vi "Get Default Data from TD.vi"(8 "error in (no error)":errorcluster, 10 "Type Descriptor":refnum<class "TD.lvclass">) -> (0 "error out":errorcluster, 2 "Default VData":refnum<class "variant.lvclass">)   [LabVIEW 2020, in "variant.lvlib" / "variant.lvclass"]
doc: "Returns default data of the type defined by the TD. This VI calls itself recursively.\n\nThis VI is <b>Reentrant</b>"
uses:
  variant.lvclass
  variant.lvclass/variant.ctl
  <userlib>/_OpenG.lib/error/error.llb/openg_error.lvlib
  TD.lvclass
  Bytes/Bytes.lvclass
  DataString/DataString.lvclass
  C:/projects/OpenG-Variant-Data-Library/source/library/Bytes/Bytes.lvclass
  C:/projects/OpenG-Variant-Data-Library/source/library/LVData/DataString/DataString.lvclass
panel:
  # "Please visit http://www.OpenG.org to learn about the\nOpen Source LabVIEW software movement.\n\nNOTICE -- YOU MUST LEAVE THIS NOTICE IN PLACE.  PER THE TERMS OF THE LICENSE BELOW, YOU MAY SUBLICENSE THIS SOFTWARE \nIN ANY WAY THAT DOES NOT CONFLICT WITH THIS LICENSE.\n\n### BSD License (http://www.opensource.org/licenses/bsd-license.php) Begin ###\n \nCopyright (c) 2002, Jean-Pierre Drolet <drolet_jp@hotmail.com>\nCopyright (c) 2002-2006, Jim Kring <jim@jimkring.com>\nCopyright (c) 2011, Jonathon Green <jg@jgcode.net>\n\nAll rights reserved.\n\nRedistribution and use in source and binary forms, with or without modification, are permitted provided that the following conditions are met:\n\n    * Redistributions of source code must retain the above copyright notice, this list of conditions and the following disclaimer.\n    * Redistributions in binary form must reproduce the above copyright notice, this list of conditions and the following disclaimer in the \n       documentation and/or other materials provided with the distribution.\n    * Neither the name of SciWare, James Kring, Inc., nor the names of its contributors may be used to endorse or promote products derived \n       from this software without specific prior written permission.\n\nTHIS SOFTWARE IS PROVIDED BY THE COPYRIGHT HOLDERS AND CONTRIBUTORS \"AS IS\" AND ANY EXPRESS OR IMPLIED WARRANTIES, \nINCLUDING, BUT NOT LIMITED TO, THE IMPLIED WARRANTIES OF MERCHANTABILITY AND FITNESS FOR A PARTICULAR PURPOSE ARE \nDISCLAIMED. IN NO EVENT SHALL THE COPYRIGHT OWNER OR CONTRIBUTORS BE LIABLE FOR ANY DIRECT, INDIRECT, INCIDENTAL,\n SPECIAL, EXEMPLARY, OR CONSEQUENTIAL DAMAGES (INCLUDING, BUT NOT LIMITED TO, PROCUREMENT OF SUBSTITUTE GOODS OR \nSERVICES; LOSS OF USE, DATA, OR PROFITS; OR BUSINESS INTERRUPTION) HOWEVER CAUSED AND ON ANY THEORY OF LIABILITY, \nWHETHER IN CONTRACT, STRICT LIABILITY, OR TORT (INCLUDING NEGLIGENCE OR OTHERWISE) ARISING IN ANY WAY OUT OF THE USE \nOF THIS SOFTWARE, EVEN IF ADVISED OF THE POSSIBILITY OF SUCH DAMAGE.\n\n### BSD License End ###"
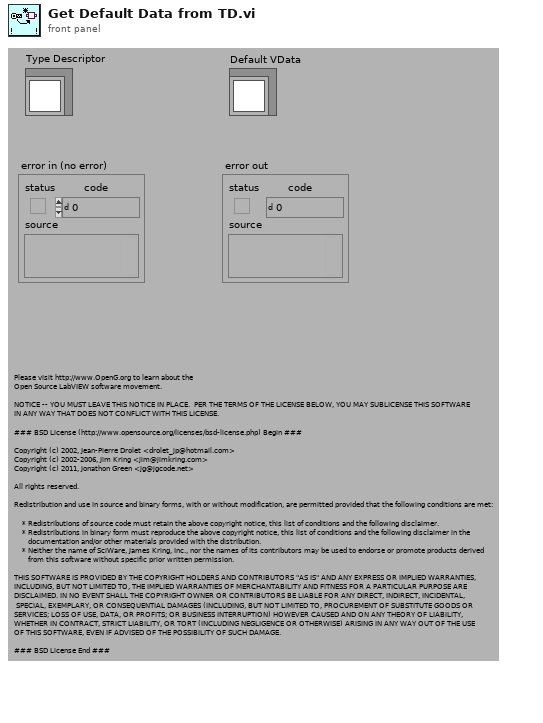
[diagram p1: front panel]
types:
  T1 = typedef "openg_variant.lvlib/Type Descriptor Enumeration.ctl" = enum8{"<Null>", "I8", "I16", "I32", "I64", "U8", "U16", "U32", "U64", "SGL", "DBL", "EXT", "CSG", "CDB", "CXT", "0x0F", "0x10", "0x11", "0x12", "0x13", "0x14", "Enum U8", "Enum U16", "Enum U32", "Enum U64", "SGL PQ", "DBL PQ", "EXT PQ", "CSG PQ", "CDB PQ", "CXT PQ", "0x1F", "0x20", "Boolean", "0x22", "0x23", "0x24", "0x25", "0x26", "0x27", "0x28", "0x29", "0x2A", "0x2B", "0x2C", "0x2D", "0x2E", "0x2F", "String", "0x31", "Path", "Pict", "0x34", "0x35", "0x36", "DAQ", "0x38", "0x39", "0x3A", "0x3B", "0x3C", "0x3D", "0x3E", "0x3F", "Array", "0x41", "0x42", "0x43", "0x44", "0x45", "0x46", "0x47", "0x48", "0x49", "0x4A", "0x4B", "0x4C", "0x4D", "0x4E", "0x4F", "Cluster", "0x51", "0x52", "Variant", "Waveform", "0x55", "0x56", "0x57", "0x58", "0x59", "0x5A", "0x5B", "0x5C", "0x5D", "0x5E", "Fixed Point", "0x60", "0x61", "0x62", "0x63", "0x64", "0x65", "0x66", "0x67", "0x68", "0x69", "0x6A", "0x6B", "0x6C", "0x6D", "0x6E", "0x6F", "Refnum", "0x71", "0x72", "Set Collection", "Map Collection"}
  T2 = typedef "openg_variant.lvlib/Waveform Subtype Enum.ctl" = enum8{"<Not a Waveform Type>", "0x01", "Analog 16-bit signed", "Analog Double-Precision", "0x04", "Analog Single Precision", "Timestamp", "Digital Data", "Digital Waveform", "Dynamic Data", "Analog Extended-Precision", "Analog 8-bit unsigned", "Analog 16-bit unsigned", "Analog 32-bit unsigned", "Analog 8-bit signed", "Analog 32-bit signed", "Analog Complex Single-Precision", "Analog Complex Double-Precision", "Analog Complex Extended Precision", "Analog 64-bit signed", "Analog 64-bit unsigned"}
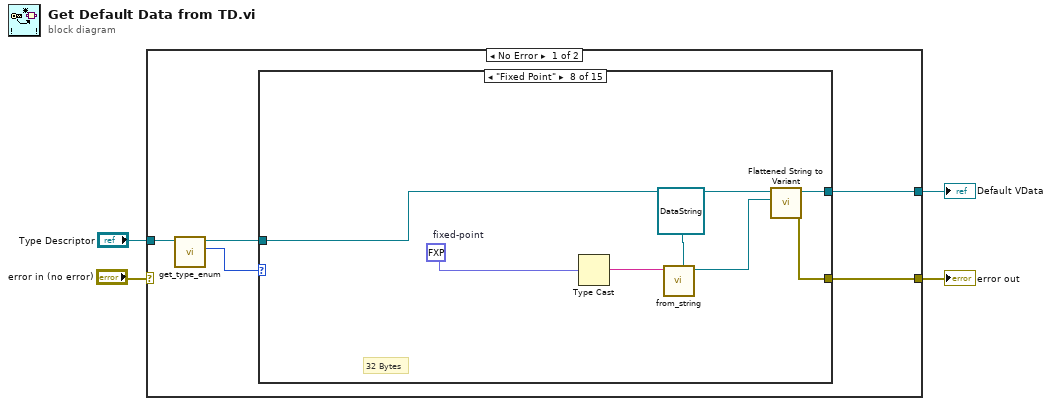
[diagram p0: block diagram]
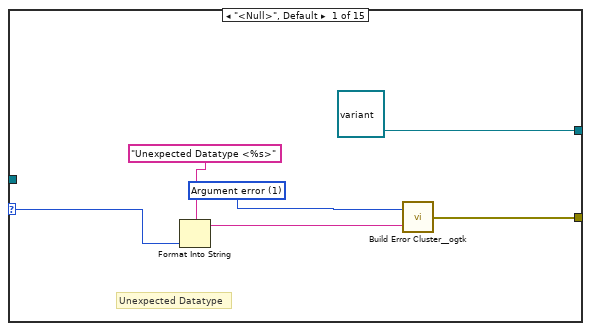
[diagram p2: hidden frame]
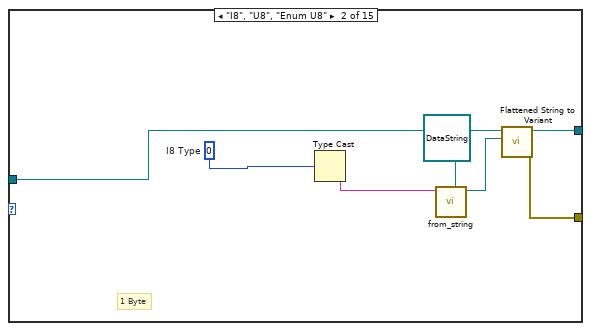
[diagram p3: hidden frame]
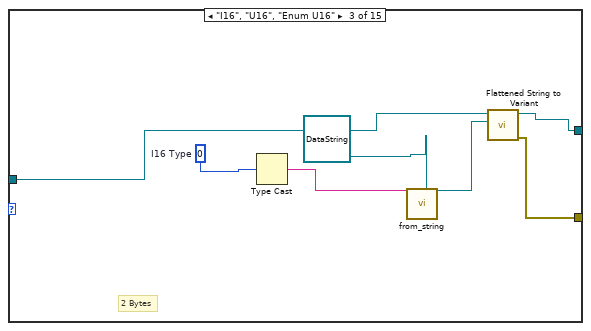
[diagram p4: hidden frame]
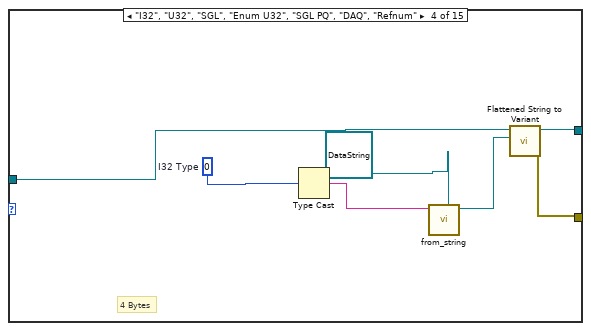
[diagram p5: hidden frame]
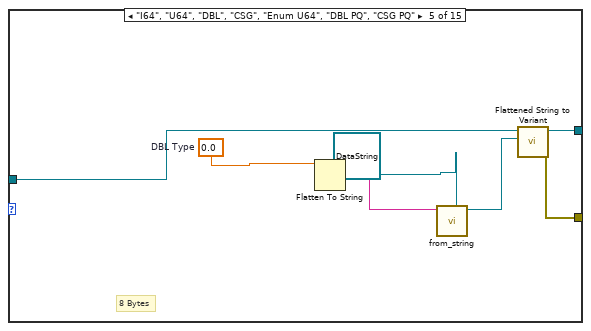
[diagram p6: hidden frame]
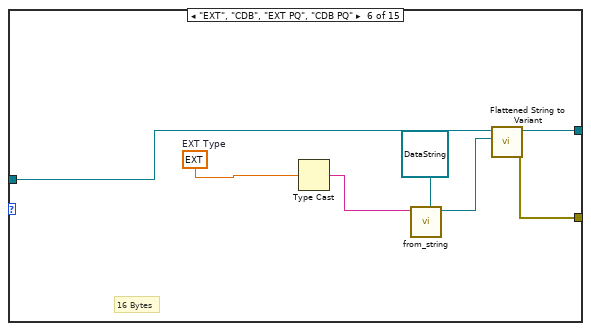
[diagram p7: hidden frame]
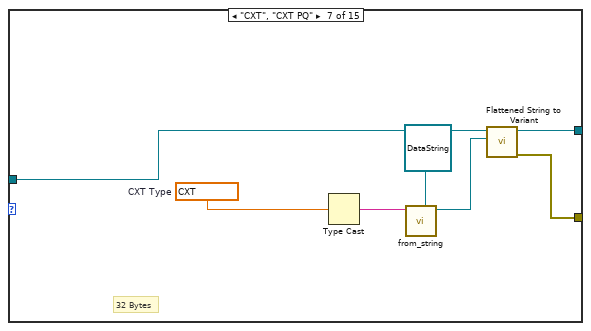
[diagram p8: hidden frame]
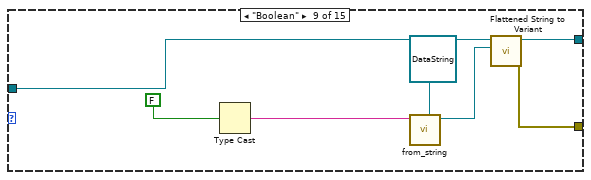
[diagram p9: hidden frame]
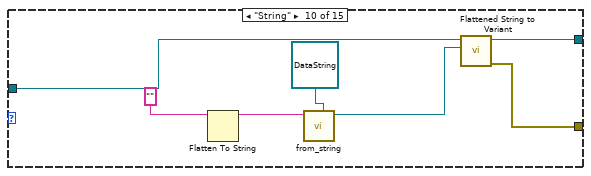
[diagram p10: hidden frame]
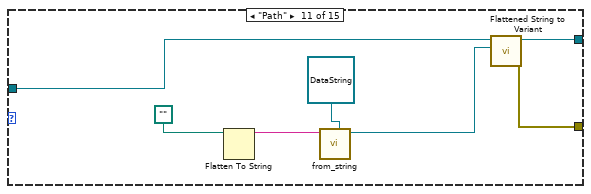
[diagram p11: hidden frame]
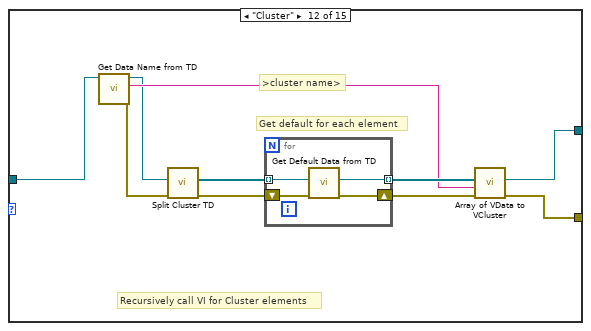
[diagram p12: hidden frame]
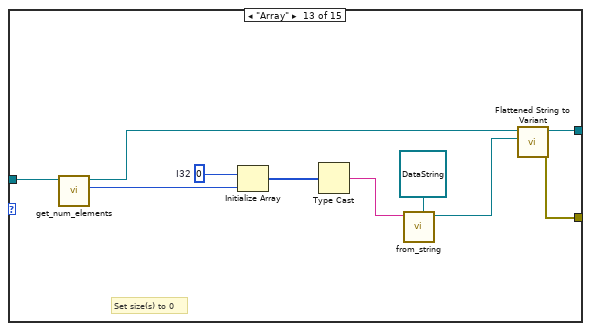
[diagram p13: hidden frame]
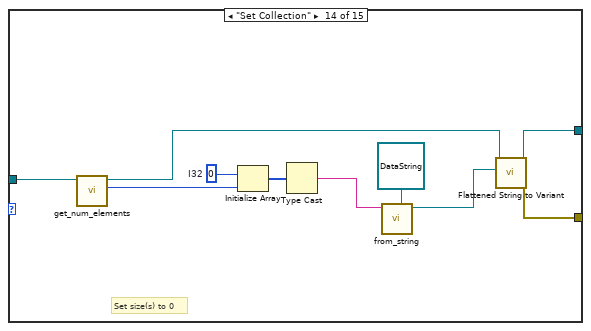
[diagram p14: hidden frame]
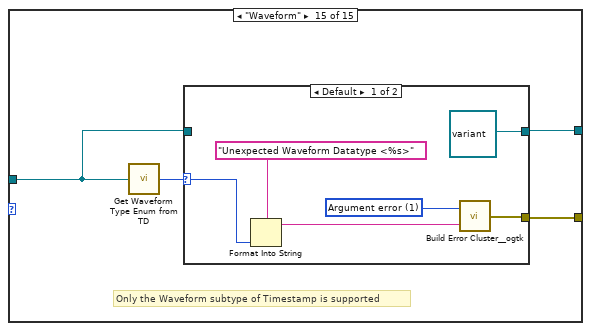
[diagram p15: hidden frame]
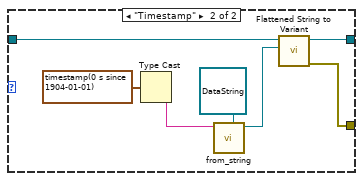
[diagram p16: hidden frame]
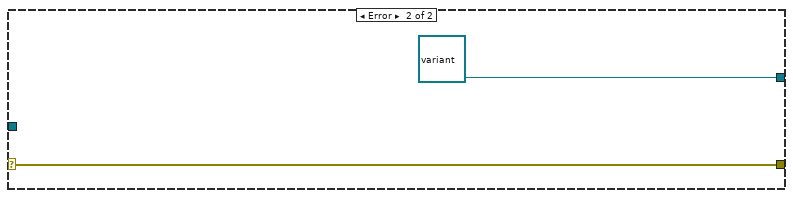
[diagram p17: hidden frame]
diagram:
  n1 = case shown="No Error" "error in (no error)" {
    selector: "error in (no error)" -> [_ w138]
    tunnel: [w9 w138] -> w2
    tunnel: "Type Descriptor" -> [w7 _]
    tunnel: [w8 refnum<class "variant.lvclass"> refnum ("Default VData")] -> w1
    frame No Error {
      n2 = call "get_type_enum.vi"("TypeDescriptor"=w7) -> ("type"=w5:T1, "TypeDescriptor out"=w6:refnum<class "TD.lvclass">)  [unwired: 9 in]
      n3 = case shown="\"Fixed Point\"" w5 {
        selector: w5 -> [w12 _ _ _ _ _ _ _ _ _ _ _ _ _ _]
        tunnel: [w11 w18 w26 w32 w39 w46 w52 w59 w67 w75 w82 w90 w101 w112 w122] -> w9
        tunnel: w6 -> [_ w17 w24 w31 w38 w45 w56 w61 w66 w74 w79 w88 w109 w117 w121]
        tunnel: [refnum<class "variant.lvclass"> refnum ("Default VData") w19 w25 w33 w40 w47 w51 w60 w68 w76 w83 w91 w103 w113 w123] -> w8
        frame "<Null>", Default {
          w13 = 1 items=["No error", "Argument error", "Memory is full", "Out of zone", "End of file", "File already open", "Generic file I/O error", "File not found", "File permission error", "Disk is full", "Duplicate path", "Too many files open", "System feature not enabled", "Resource file not found", "Cannot add resource", "Resource not found", "Image not found", "Image memory error", "Pen does not exist", "Config type invalid", "Config token not found", "Config parse error", "Config memory error", "Bad external code format", "Bad external code offset", "External code not present", "Null window", "Destroy window error", "Null menu", "Print aborted", "Bad print record", "Print driver error", "Windows error during printing", "Memory error during printing", "Print dialog error", "Generic print error", "Invalid device refnum", "Device not found", "Device parameter error", "Device unit error", "Cannot open device", "Device call aborted", "Generic error", "Cancelled by user", "Object ID too low", "Object ID too high", "Object not in heap", "Unknown heap", "Unknown object (invalid DefProc)", "Unknown object (DefProc not in table)", "Message out of range", "Invalid (null) method", "Unknown message", "Manager call not supported", "Bad address", "Network operation in progress", "Network operation timed out", "Connection is busy", "Network attribute not supported", "Network error", "Address in use", "System out of memory", "Connection aborted", "Connection refused", "Not connected", "Already connected", "Connection closed", "Initialization error (interapplication manager)", "Bad occurrence", "Wait on unbound occurrence handler", "Occurrence queue overflow", "Datalog type conflict", "Unused", "Unrecognized type (interapplication manager)", "Memory corrupt", "Failed to make temporary DLL", "Old CIN version", "Drag socket not found", "Failed to load drop-object", "Failed to register OLE object", "Failed to release OLE object", "Format specifier type mismatch", "Unknown format specifier", "Too few format specifiers", "Too many format specifiers", "Scan failed", "Newer CIN version", "Error converting to variant", "Runtime menu error", "Password tampered", "Variant attribute not found", "Incompatible variant data type", "Event data is not available", "Event Store is not present", "Occurrence is not found", "Event Queue is not created", "Event info is not available", "Refnum passed is NULL", "Error retrieving Class GUID", "Error retrieving CoClass GUID", "Error retrieving TypeLib GUID.", "Bad built application magic bytes.", "Specific driver is different from the specific driver associated with the Logical Name.", "There is no session opened to the class driver.", "Max Error", "MAX - Error with config objects", "MAX - Error loading configuration", "MAX - Group not supported"]
          # "Unexpected Datatype"
          n4 = Format Into String(format string="Unexpected Datatype <%s>" ("Format String"), w12) -> (resulting string=w15:string)  [unwired: 2 in, 1 out]
          n5 = call <userlib>:"Build Error Cluster__ogtk.vi"("String to Prepend to source (\"\")"=w15, "code"=w13) -> ("error out"=w11:errorcluster)
        }
        frame "I8", "U8", "Enum U8" {
          w22 = i8 0  # I8 Type
          # "1 Byte"
          n6 = Type Cast(x=w22) -> (*(type *) &x=w16:string)  [unwired: 1 in]
          n7 = call "from_string.vi"("type"=refnum<class "DataString.lvclass"> refnum ("data"), "string_data"=w16) -> ("Bytes out"=w21:refnum<class "DataString.lvclass">)  [unwired: 9 in]
          n8 = call "Flattened String to Variant.vi"("data"=w21, "type"=w17) -> ("error out"=w18:errorcluster, "variant out"=w19:refnum<class "variant.lvclass">)  [unwired: 8 in]
        }
        frame "I16", "U16", "Enum U16" {
          w29 = i16 0  # I16 Type
          # "2 Bytes"
          n9 = Type Cast(x=w29) -> (*(type *) &x=w23:string)  [unwired: 1 in]
          n10 = call "from_string.vi"("type"=refnum<class "DataString.lvclass"> refnum ("data"), "string_data"=w23) -> ("Bytes out"=w28:refnum<class "DataString.lvclass">)  [unwired: 9 in]
          n11 = call "Flattened String to Variant.vi"("data"=w28, "type"=w24) -> ("error out"=w26:errorcluster, "variant out"=w25:refnum<class "variant.lvclass">)  [unwired: 8 in]
        }
        frame "I32", "U32", "SGL", "Enum U32", "SGL PQ", "DAQ", "Refnum" {
          w36 = 0  # I32 Type
          # "4 Bytes"
          n12 = Type Cast(x=w36) -> (*(type *) &x=w30:string)  [unwired: 1 in]
          n13 = call "from_string.vi"("type"=refnum<class "DataString.lvclass"> refnum ("data"), "string_data"=w30) -> ("Bytes out"=w35:refnum<class "DataString.lvclass">)  [unwired: 9 in]
          n14 = call "Flattened String to Variant.vi"("data"=w35, "type"=w31) -> ("error out"=w32:errorcluster, "variant out"=w33:refnum<class "variant.lvclass">)  [unwired: 8 in]
        }
        frame "I64", "U64", "DBL", "CSG", "Enum U64", "DBL PQ", "CSG PQ" {
          w43 = 0.0  # DBL Type
          # "8 Bytes"
          n15 = Flatten To String(anything=w43) -> (data string=w37:string)  [unwired: 3 in, 2 out]
          n16 = call "from_string.vi"("type"=refnum<class "DataString.lvclass"> refnum ("data"), "string_data"=w37) -> ("Bytes out"=w42:refnum<class "DataString.lvclass">)  [unwired: 9 in]
          n17 = call "Flattened String to Variant.vi"("data"=w42, "type"=w38) -> ("error out"=w39:errorcluster, "variant out"=w40:refnum<class "variant.lvclass">)  [unwired: 8 in]
        }
        frame "EXT", "CDB", "EXT PQ", "CDB PQ" {
          w50 = ext 0.0  # EXT Type
          # "16 Bytes"
          n18 = Type Cast(x=w50) -> (*(type *) &x=w44:string)  [unwired: 1 in]
          n19 = call "from_string.vi"("type"=refnum<class "DataString.lvclass"> refnum ("data"), "string_data"=w44) -> ("Bytes out"=w49:refnum<class "DataString.lvclass">)  [unwired: 9 in]
          n20 = call "Flattened String to Variant.vi"("data"=w49, "type"=w45) -> ("error out"=w46:errorcluster, "variant out"=w47:refnum<class "variant.lvclass">)  [unwired: 8 in]
        }
        frame "CXT", "CXT PQ" {
          w57 = cxt 0.0+0.0i  # CXT Type
          # "32 Bytes"
          n21 = Type Cast(x=w57) -> (*(type *) &x=w53:string)  [unwired: 1 in]
          n22 = call "from_string.vi"("type"=refnum<class "DataString.lvclass"> refnum ("data"), "string_data"=w53) -> ("Bytes out"=w55:refnum<class "DataString.lvclass">)  [unwired: 9 in]
          n23 = call "Flattened String to Variant.vi"("data"=w55, "type"=w56) -> ("error out"=w52:errorcluster, "variant out"=w51:refnum<class "variant.lvclass">)  [unwired: 8 in]
        }
        frame "Fixed Point" {
          w64 = fxp<+/-,32,16> 0.0  # fixed-point
          # "32 Bytes"
          n24 = Type Cast(x=w64) -> (*(type *) &x=w58:string)  [unwired: 1 in]
          n25 = call "from_string.vi"("type"=refnum<class "DataString.lvclass"> refnum ("data"), "string_data"=w58) -> ("Bytes out"=w63:refnum<class "DataString.lvclass">)  [unwired: 9 in]
          n26 = call "Flattened String to Variant.vi"("data"=w63, "type"=w61) -> ("error out"=w59:errorcluster, "variant out"=w60:refnum<class "variant.lvclass">)  [unwired: 8 in]
        }
        frame "Boolean" {
          n27 = Type Cast(x=FALSE ("status")) -> (*(type *) &x=w65:string)  [unwired: 1 in]
          n28 = call "from_string.vi"("type"=refnum<class "DataString.lvclass"> refnum ("data"), "string_data"=w65) -> ("Bytes out"=w70:refnum<class "DataString.lvclass">)  [unwired: 9 in]
          n29 = call "Flattened String to Variant.vi"("data"=w70, "type"=w66) -> ("error out"=w67:errorcluster, "variant out"=w68:refnum<class "variant.lvclass">)  [unwired: 8 in]
        }
        frame "String" {
          n30 = Flatten To String(anything="") -> (data string=w73:string)  [unwired: 3 in, 2 out]
          n31 = call "from_string.vi"("type"=refnum<class "DataString.lvclass"> refnum ("data"), "string_data"=w73) -> ("Bytes out"=w77:refnum<class "DataString.lvclass">)  [unwired: 9 in]
          n32 = call "Flattened String to Variant.vi"("data"=w77, "type"=w74) -> ("error out"=w75:errorcluster, "variant out"=w76:refnum<class "variant.lvclass">)  [unwired: 8 in]
        }
        frame "Path" {
          n33 = Flatten To String(anything=path "") -> (data string=w80:string)  [unwired: 3 in, 2 out]
          n34 = call "from_string.vi"("type"=refnum<class "DataString.lvclass"> refnum ("data"), "string_data"=w80) -> ("Bytes out"=w84:refnum<class "DataString.lvclass">)  [unwired: 9 in]
          n35 = call "Flattened String to Variant.vi"("data"=w84, "type"=w79) -> ("error out"=w82:errorcluster, "variant out"=w83:refnum<class "variant.lvclass">)  [unwired: 8 in]
        }
        frame "Cluster" {
          # "Get default for each element"
          # "Recursively call VI for Cluster elements"
          # ">cluster name>"
          n36 = call "Get Data Name from TD.vi"("TypeDescriptor"=w88) -> ("error"=w87:errorcluster, "name"=w92:string, "TypeDescriptor out"=w89:refnum<class "TD.lvclass">)  [unwired: 8 in]
          n37 = call "Split Cluster TD.vi"("error in (no error)"=w87, "Cluster TD"=w89) -> ("error out"=w86:errorcluster, "element TypeDescriptors"=w94:refnum<class "TD.lvclass">[])  [unwired: 8 in]
          n38 = for {
            tunnel: w94 -> [w99] mode=indexing
            shift-right: [w97] -> w93
            shift-left: w86 -> [w98]
            tunnel: [w96] -> w95 mode=indexing
            n39 = call "Get Default Data from TD.vi"("error in (no error)"=w98, "Type Descriptor"=w99) -> ("error out"=w97:errorcluster, "Default VData"=w96:refnum<class "variant.lvclass">)  [unwired: 8 in]
          }
          n40 = call "Array of VData to VCluster.vi"("error in (no error)"=w93, "Cluster Name"=w92, "Array"=w95) -> ("error out"=w90:errorcluster, "VCluster"=w91:refnum<class "variant.lvclass">)  [unwired: 7 in]
        }
        frame "Array" {
          w108 = 0  # I32
          # "Set size(s) to 0"
          n41 = call "get_num_elements.vi"("TypeDescriptor"=w109) -> ("num_element"=w106:i32, "TypeDescriptor out"=w102:refnum<class "TD.lvclass">)  [unwired: 9 in]
          n42 = Initialize Array(w108, w106) -> (w107:i32[])
          n43 = Type Cast(x=w107) -> (*(type *) &x=w100:string)  [unwired: 1 in]
          n44 = call "from_string.vi"("type"=refnum<class "DataString.lvclass"> refnum ("data"), "string_data"=w100) -> ("Bytes out"=w105:refnum<class "DataString.lvclass">)  [unwired: 9 in]
          n45 = call "Flattened String to Variant.vi"("data"=w105, "type"=w102) -> ("error out"=w101:errorcluster, "variant out"=w103:refnum<class "variant.lvclass">)  [unwired: 8 in]
        }
        frame "Set Collection" {
          w119 = 0  # I32
          # "Set size(s) to 0"
          n46 = call "get_num_elements.vi"("TypeDescriptor"=w117) -> ("num_element"=w116:i32, "TypeDescriptor out"=w111:refnum<class "TD.lvclass">)  [unwired: 9 in]
          n47 = Initialize Array(w119, w116) -> (w118:i32[])
          n48 = Type Cast(x=w118) -> (*(type *) &x=w110:string)  [unwired: 1 in]
          n49 = call "from_string.vi"("type"=refnum<class "DataString.lvclass"> refnum ("data"), "string_data"=w110) -> ("Bytes out"=w115:refnum<class "DataString.lvclass">)  [unwired: 9 in]
          n50 = call "Flattened String to Variant.vi"("data"=w115, "type"=w111) -> ("error out"=w112:errorcluster, "variant out"=w113:refnum<class "variant.lvclass">)  [unwired: 8 in]
        }
        frame "Waveform" {
          # "Only the Waveform subtype of Timestamp is supported"
          n51 = call "Get Waveform Type Enum from TD.vi"("Type Descriptor"=w121) -> ("Waveform Subtype Enum"=w120:T2)  [unwired: 4 in]
          n52 = case shown="Default" w120 {
            selector: w120 -> [w125 _]
            tunnel: [refnum<class "variant.lvclass"> refnum ("Default VData") w136] -> w123
            tunnel: [w126 w135] -> w122
            tunnel: w121 -> [_ w134]
            frame Default {
              w127 = 1 items=["No error", "Argument error", "Memory is full", "Out of zone", "End of file", "File already open", "Generic file I/O error", "File not found", "File permission error", "Disk is full", "Duplicate path", "Too many files open", "System feature not enabled", "Resource file not found", "Cannot add resource", "Resource not found", "Image not found", "Image memory error", "Pen does not exist", "Config type invalid", "Config token not found", "Config parse error", "Config memory error", "Bad external code format", "Bad external code offset", "External code not present", "Null window", "Destroy window error", "Null menu", "Print aborted", "Bad print record", "Print driver error", "Windows error during printing", "Memory error during printing", "Print dialog error", "Generic print error", "Invalid device refnum", "Device not found", "Device parameter error", "Device unit error", "Cannot open device", "Device call aborted", "Generic error", "Cancelled by user", "Object ID too low", "Object ID too high", "Object not in heap", "Unknown heap", "Unknown object (invalid DefProc)", "Unknown object (DefProc not in table)", "Message out of range", "Invalid (null) method", "Unknown message", "Manager call not supported", "Bad address", "Network operation in progress", "Network operation timed out", "Connection is busy", "Network attribute not supported", "Network error", "Address in use", "System out of memory", "Connection aborted", "Connection refused", "Not connected", "Already connected", "Connection closed", "Initialization error (interapplication manager)", "Bad occurrence", "Wait on unbound occurrence handler", "Occurrence queue overflow", "Datalog type conflict", "Unused", "Unrecognized type (interapplication manager)", "Memory corrupt", "Failed to make temporary DLL", "Old CIN version", "Drag socket not found", "Failed to load drop-object", "Failed to register OLE object", "Failed to release OLE object", "Format specifier type mismatch", "Unknown format specifier", "Too few format specifiers", "Too many format specifiers", "Scan failed", "Newer CIN version", "Error converting to variant", "Runtime menu error", "Password tampered", "Variant attribute not found", "Incompatible variant data type", "Event data is not available", "Event Store is not present", "Occurrence is not found", "Event Queue is not created", "Event info is not available", "Refnum passed is NULL", "Error retrieving Class GUID", "Error retrieving CoClass GUID", "Error retrieving TypeLib GUID.", "Bad built application magic bytes.", "Specific driver is different from the specific driver associated with the Logical Name.", "There is no session opened to the class driver.", "Max Error", "MAX - Error with config objects", "MAX - Error loading configuration", "MAX - Group not supported"]
              n53 = Format Into String(format string="Unexpected Waveform Datatype <%s>" ("Format String"), w125) -> (resulting string=w129:string)  [unwired: 2 in, 1 out]
              n54 = call <userlib>:"Build Error Cluster__ogtk.vi"("String to Prepend to source (\"\")"=w129, "code"=w127) -> ("error out"=w126:errorcluster)
            }
            frame "Timestamp" {
              n55 = Type Cast(x=timestamp(0 s since 1904-01-01) ("Time Stamp")) -> (*(type *) &x=w132:string)  [unwired: 1 in]
              n56 = call "from_string.vi"("type"=refnum<class "DataString.lvclass"> refnum ("data"), "string_data"=w132) -> ("Bytes out"=w130:refnum<class "DataString.lvclass">)  [unwired: 9 in]
              n57 = call "Flattened String to Variant.vi"("data"=w130, "type"=w134) -> ("error out"=w135:errorcluster, "variant out"=w136:refnum<class "variant.lvclass">)  [unwired: 8 in]
            }
          }
        }
      }
    }
    frame Error {
    }
  }
  "error out" <- w2
  "Default VData" <- w1
